vi "Configure.vi"(8 "error in (no error)":errorcluster, 11 "Mag Lab Measure Interface in":refnum<class "MagLabGraph.lvclass">) -> (0 "error out":errorcluster, 3 "Mag Lab Measure Interface out":refnum<class "MagLabGraph.lvclass">)   [LabVIEW 2015, in "MagLabGraph.lvclass"]
uses:
  MagLabGraph.lvclass
  Mag Lab Measure Interface/Mag Lab Measure UI.lvclass
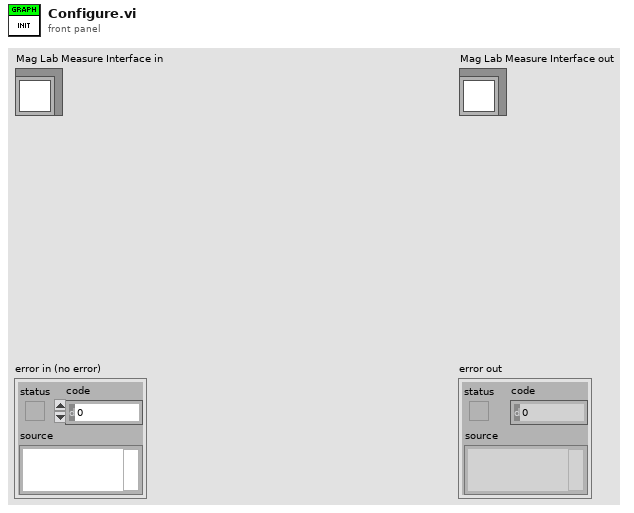
[diagram p1: front panel]
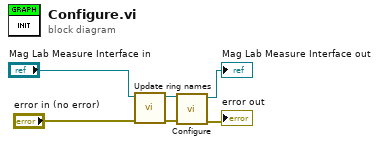
[diagram p0: block diagram]
diagram:
  n1 = call "Update ring names.vi"("error in (no error)"="error in (no error)", "MagLabGraph in"="Mag Lab Measure Interface in") -> ("error out"=w4:errorcluster, "MagLabGraph out"=w2:refnum<class "MagLabGraph.lvclass">)  [unwired: 8 in]
  n2 = call-parent "Configure.vi"("error in (no error)"=w4, "Mag Lab Measure Interface in"=w2) -> ("error out"=→"error out":errorcluster, "Mag Lab Measure Interface out"=→"Mag Lab Measure Interface out":refnum<class "MagLabGraph.lvclass">)  [unwired: 8 in]
